vi "fgv_cam_config.vi"(7 "cmd":enum16{"read", "write"}(ring), 11 "camera cfg":cluster{"Port":T1, "Camera file":path}={"Port"="cam2", "Camera file"=path "C:/AGV/Config/camera/C920.icd"}) -> (3 "camera cfg out":cluster{"Port":T1, "Camera file":path}={"Port"="cam2", "Camera file"=path "C:/AGV/Config/camera/C920.icd"})   [LabVIEW 2019]
uses:
  <vilib>/userDefined/High Color/IMAQdx.ctl
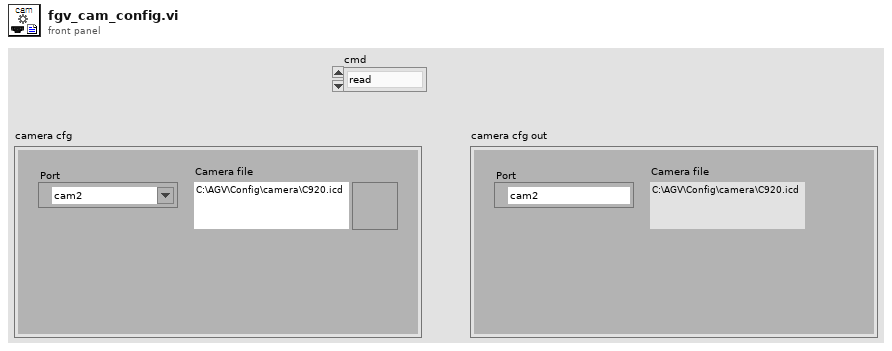
[diagram p1: front panel]
types:
  T1 = typedef "IMAQdx.ctl" = refnum<k21>
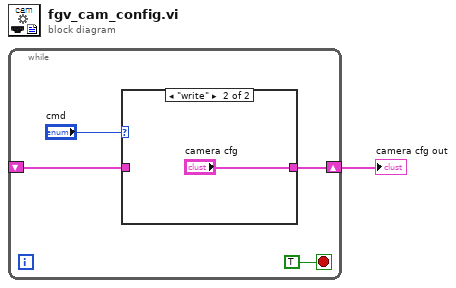
[diagram p0: block diagram]
diagram:
  n1 = while {
    shift-right: [w3] -> w1
    shift-left: _ -> [w2]
    stop <- TRUE stop-if-true
    n2 = case shown="\"write\"" "cmd" {
      tunnel: [w6 "camera cfg"] -> w3
      tunnel: w2 -> [w6 _]
      frame "read", Default {
      }
      frame "write" {
      }
    }
  }
  "camera cfg out" <- w1
